vi "HHMI - Count U8 with set rollover.vi"(6 "set to zero when count =":u8=255, 7 "Reset?":bool, 10 "Increment?":bool) -> (2 "total # counted\n(Reset occurs \nprior to Increment)":u8)   [LabVIEW 2013]
doc: "Counts up. Reset returns count to zero. Increment occurs after Reset."
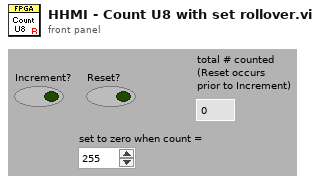
[diagram p1: front panel]
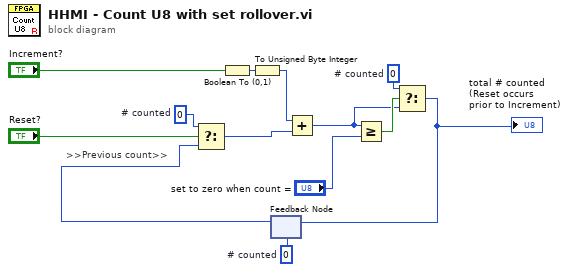
[diagram p0: block diagram]
diagram:
  w6 = u8 0  # # counted
  w10 = u8 0  # # counted
  w13 = u8 0  # # counted
  # ">>Previous count>>"
  n1 = Boolean To (0,1)(Boolean="Increment?") -> (0, 1=w3:i16)
  n2 = To Unsigned Byte Integer(number=w3) -> (unsigned 8bit integer=w1:u8)
  n3 = feedback #1(w13) -> (w11:u8)
  n4 = Select(t=w10, s="Reset?", f=w11) -> (s? t:f=w5:u8)
  n5 = Add(x=w1, y=w5) -> (x+y=w2:u8)
  n6 = Greater Or Equal?(x=w2, y="set to zero when count =") -> (x >= y?=w8:bool)
  n7 = Select(t=w6, s=w8, f=w2) -> (s? t:f=w7:u8)
  "total # counted\n(Reset occurs \nprior to Increment)" <- w7
  n8 = feedback-in #1(w7) -> ()
